vi "ADCP_Generate_Checksum_Processed_Packet.vi"(8 "error in (no error)":errorcluster, 10 "Processed Packet In":u8[](array[numeric]), 11 "ADCP in":refnum<class "ADCP.lvclass">) -> (0 "error out":errorcluster, 1 "Checksum":u8, 2 "Processed Packet Out":u8[](array[numeric]), 3 "ADCP out":refnum<class "ADCP.lvclass">)   [LabVIEW 2017, in "ADCP.lvclass"]
uses:
  ADCP.lvclass
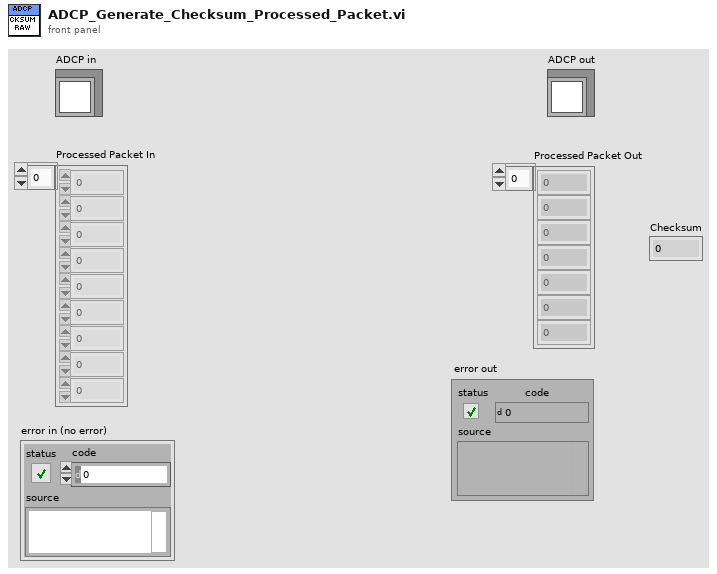
[diagram p1: front panel]
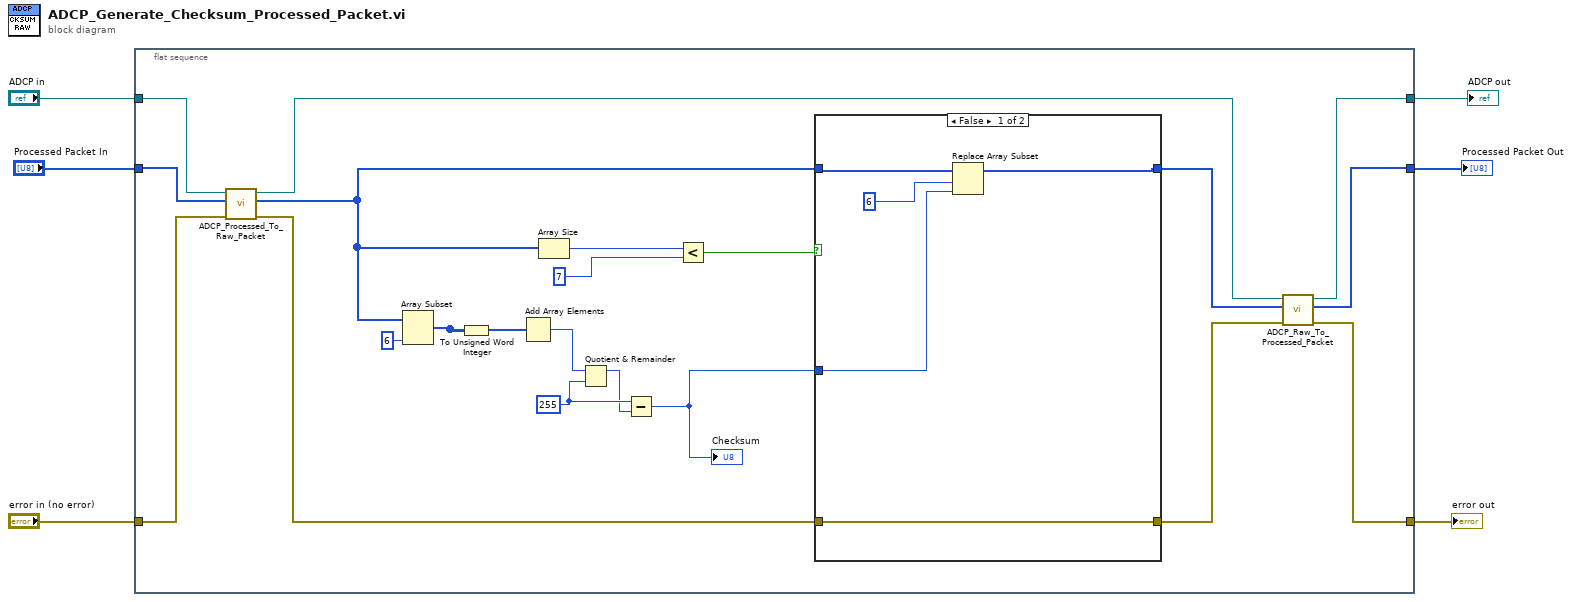
[diagram p0: block diagram]
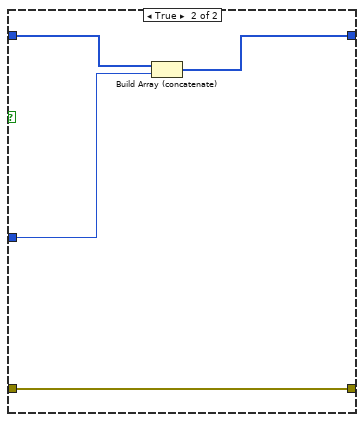
[diagram p2: hidden frame]
diagram:
  n1 = flat-sequence {
    tunnel: "error in (no error)" -> [w18]
    tunnel: [w10] -> w5
    tunnel: "ADCP in" -> [w19]
    tunnel: [w13] -> w3
    tunnel: "Processed Packet In" -> [w20]
    tunnel: [w12] -> w1
    frame #0 {
      w9 = u8 255 ("y")
      n2 = call "ADCP_Processed_To_Raw_Packet.vi"("error in (no error)"=w18, "Processed Packet"=w20, "ADCP in"=w19) -> ("error out"=w17:errorcluster, "Raw Packet"=w16:u8[], "ADCP out"=w14:refnum<class "ADCP.lvclass">)  [unwired: 6 in]
      n3 = Array Subset(array=w16, length=6) -> (w25:u8[])  [unwired: 1 in]
      n4 = To Unsigned Word Integer(number=w25) -> ()  [unwired: 1 out]
      n5 = Add Array Elements(numeric array=w25) -> (sum=w24:u8)
      n6 = Array Size(array=w16) -> (size(s)=w23:i32)
      n7 = Quotient & Remainder(x=w24, y=w9) -> (x-y*floor(x/y)=w8:u8)  [unwired: 1 out]
      n8 = Subtract(x=w9, y=w8) -> (x-y=w7:u8)
      "Checksum" <- w7
      n9 = Less?(x=w23, y=7) -> (x < y?=w21:bool)
      n10 = case shown="False" w21 {
        tunnel: w17 -> [w31 w35]
        tunnel: [w31 w35] -> w11
        tunnel: w16 -> [w30 w34]
        tunnel: w7 -> [w28 w33]
        tunnel: [w27 w32] -> w15
        frame False {
          n11 = Replace Array Subset(array=w30, new element=w28, index=6) -> (w27:u8[])
        }
        frame True {
          n12 = Build Array (concatenate)(w34, w33) -> (w32:u8[])
        }
      }
      n13 = call "ADCP_Raw_To_Processed_Packet.vi"("error in (no error)"=w11, "Raw Packet"=w15, "ADCP in"=w14) -> ("error out"=w10:errorcluster, "Processed Packet"=w12:u8[], "ADCP out"=w13:refnum<class "ADCP.lvclass">)  [unwired: 6 in]
    }
  }
  "ADCP out" <- w3
  "error out" <- w5
  "Processed Packet Out" <- w1
